vi "test2.vi"(8 "错误输入（无错误）":errorcluster, 10 "基地址":u32=1048576 format="%.0x", 11 "VISA资源名称":refnum<visa-resource-name>) -> (0 "错误输出":errorcluster, 2 "数据":u32[](array[numeric]), 3 "VISA资源名称输出":refnum<visa-resource-name>)   [LabVIEW 2012]
uses:
  <vilib>/Instr/_visa.llb/VISA Register Access Address Space.ctl
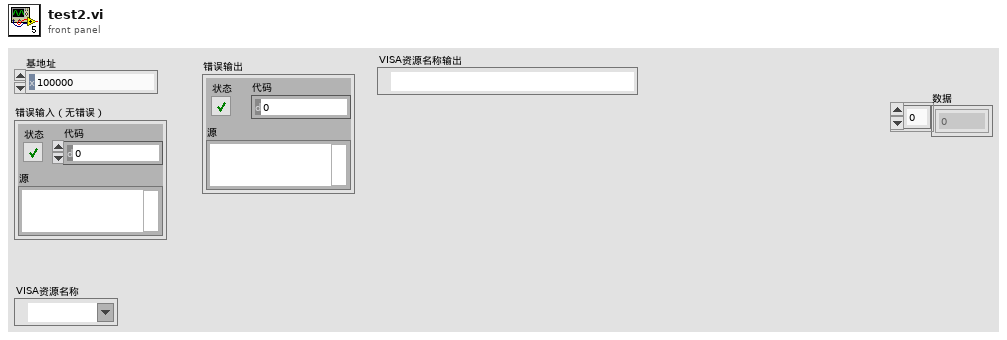
[diagram p1: front panel]
types:
  T1 = typedef "VISA Register Access Address Space.ctl" = u16
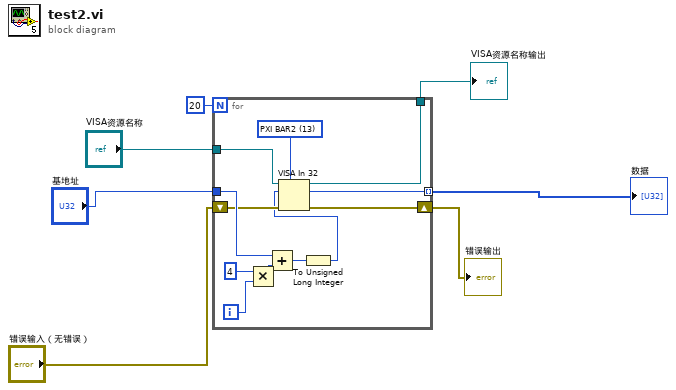
[diagram p0: block diagram]
diagram:
  n1 = for {
    N: 20 -> [_]
    tunnel: "基地址" -> [w16]
    tunnel: [w15] -> w2 mode=indexing
    tunnel: "VISA资源名称" -> [w14]
    shift-right: [w11] -> w4
    shift-left: "错误输入（无错误）" -> [w12]
    tunnel: [w10] -> w3
    i -> [w18]
    w13 = T1 13 items=["VXI/VME A16"=1, "VXI/VME A24"=2, "VXI/VME A32"=3, "VXI/VME A64"=4, "PXI内存分配"=9, "PXI配置"=10, "PXI BAR0"=11, "PXI BAR1"=12, "PXI BAR2"=13, "PXI BAR3"=14, "PXI BAR4"=15, "PXI BAR5"=16] ("Address Space")
    n2 = Multiply(x=4, y=w18) -> (x*y=w19:i32)
    n3 = Add(x=w16, y=w19) -> (x+y=w9:u32)
    n4 = To Unsigned Long Integer(number=w9) -> (unsigned 32bit integer=w8:u32)
    n5 = VISA In 32(7:w13, 8:w12, 10:w8, 11:w14) -> (0:w11:errorcluster, 2:w15:u32, 3:w10:refnum<visa-resource-name>)
  }
  "错误输出" <- w4
  "VISA资源名称输出" <- w3
  "数据" <- w2
